vi "Write Unit ID.vi"(8 "error in (no error)":errorcluster, 10 "unit ID":u8, 11 "transmission data unit in":refnum<class "Transmission Data Unit.lvclass">) -> (0 "error out":errorcluster, 3 "transmission data unit out":refnum<class "Transmission Data Unit.lvclass">)   [LabVIEW 2020, in "SubVIs.lvlib" / "Transmission Data Unit.lvclass"]
doc: "Sets the unit ID of the device."
uses:
  <vilib>/Modbus/subvis/Transmission Data Unit (ADU)/Transmission Data Unit/Transmission Data Unit.lvclass
  <vilib>/Modbus/subvis/Transmission Data Unit (ADU)/Transmission Data Unit/Transmission Data Unit.lvclass/Transmission Data Unit.ctl
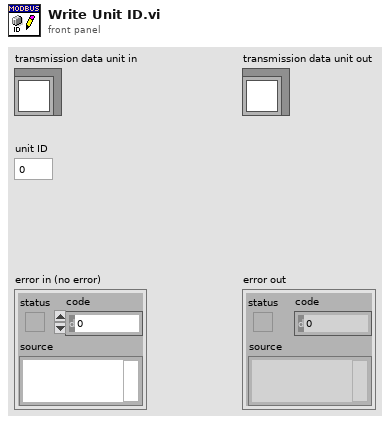
[diagram p1: front panel]
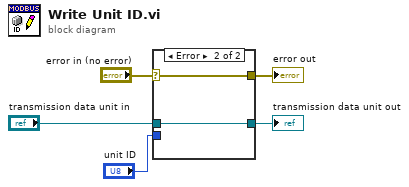
[diagram p0: block diagram]
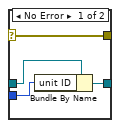
[diagram p2: hidden frame]
diagram:
  n1 = case shown="Error" "error in (no error)" {
    selector: "error in (no error)" -> [w6 w10]
    tunnel: "transmission data unit in" -> [w9 w11]
    tunnel: [w8 w11] -> w4
    tunnel: "unit ID" -> [w7 _]
    tunnel: [w6 w10] -> w1
    frame No Error {
      n2 = Bundle By Name(cluster=w9, "unit ID"=w7) -> (w8:refnum<class "Transmission Data Unit.lvclass">)
    }
    frame Error {
    }
  }
  "error out" <- w1
  "transmission data unit out" <- w4
